vi "OFBS_readTrainingData.vi"(6 "Use equal number of trials?":bool, 8 "error in (no error)":errorcluster, 9 "ControlRefs":T1, 10 "NumberOfChannels":i32, 11 "OFBS class in":refnum<class "OptFreqBandsSearch.lvclass">) -> (0 "error out":errorcluster, 2 "Num of Trials of each Class":i32[](array[numeric]), 3 "OFBS class out":refnum<class "OptFreqBandsSearch.lvclass">)   [LabVIEW 2016, in "Optimal Frequency Bands Search.lvlib" / "OptFreqBandsSearch.lvclass"]
doc: "Метод, реализующий чтение обучающих данных (проб) из xml файла"
uses:
  OptFreqBandsSearch.lvclass
  OptFreqBandsSearch.lvclass/OptFreqBandsSearch.ctl
  <vilib>/xml/Load XML File.vi
  <vilib>/xml/Close Reference(Node).vi
  _XML_EEG_Features/XML_EEG_Features.lvlib
  <vilib>/xml/NI_XML.lvlib
  Optimal Frequency Bands Search.lvlib
panel:
  # "This VI is a part of BCI Design library, http://www.ru-bci.org \nCopyright © 2020, Sotnikov Peter, All rights reserved. License: GNU GPLv3"
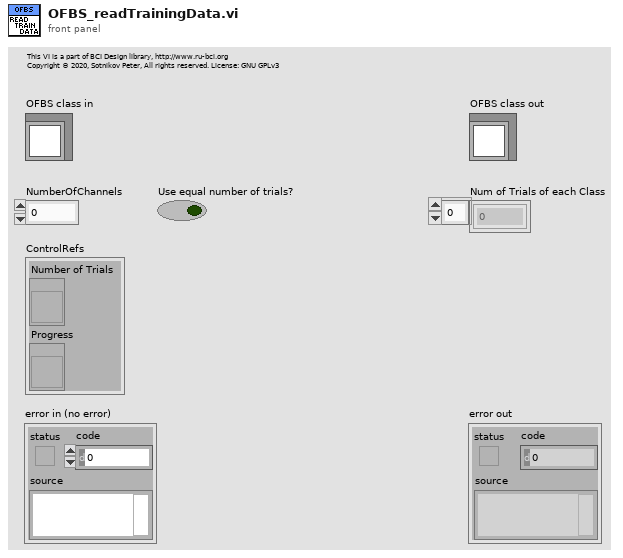
[diagram p1: front panel]
types:
  T1 = cluster{"Number of Trials":refnum<vi>, "Progress":refnum<vi>}
  T2 = typedef "XML_EEG_Features.lvlib/XML_FF_Header.ctl" = cluster{"NumberOfTrials":i32, "NumberOfClasses":i32, "FeatureVectorLength":i32, "FeatureExtractionMethod":string}
  T3 = typedef "XML_EEG_Features.lvlib/XML_FF_Trial.ctl" = cluster{"ClassLabel":string, "FeatureVector":dbl[]}
  T4 = cluster{"ClassLabel":string, "FeatureVector":dbl[][]}
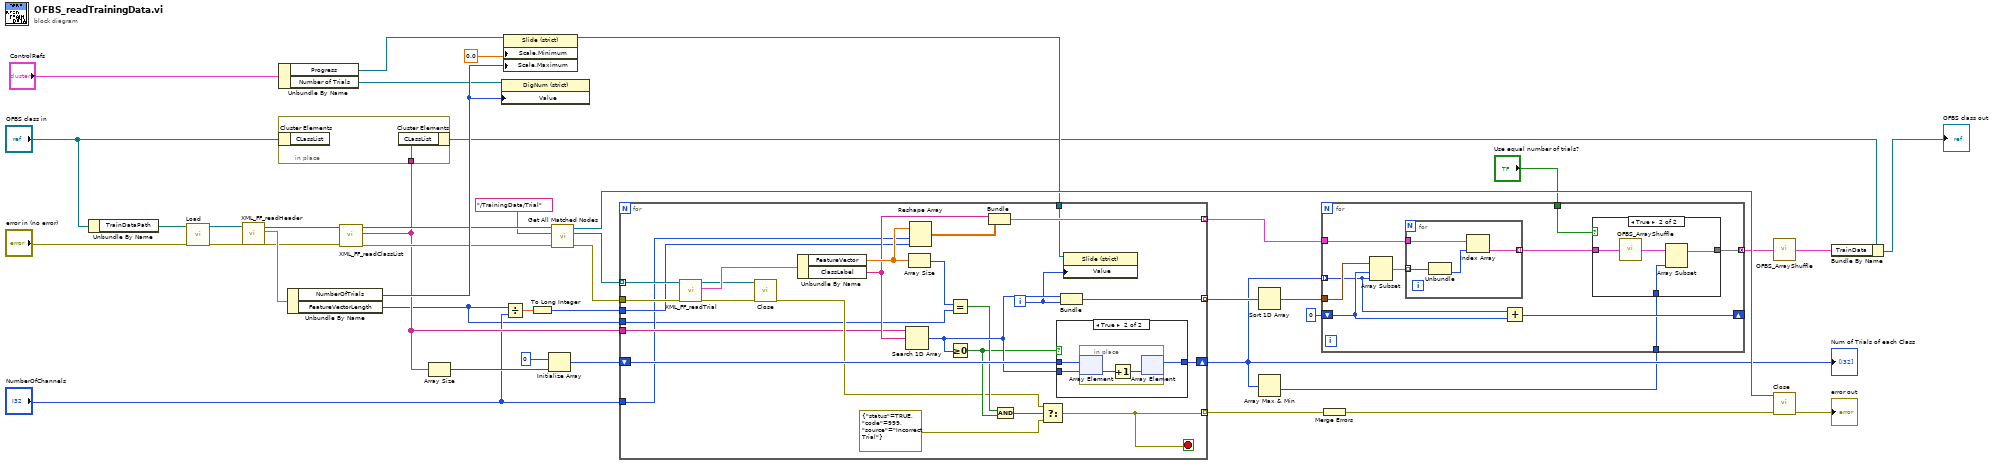
[diagram p0: block diagram]
diagram:
  n1 = Unbundle By Name("OFBS class in") -> ("TrainDataPath"=w42:path)
  n2 = call-poly <vilib>:"Load.vi"("path to XML document"=w42, "error in (no error)"="error in (no error)") -> ("DOM document out"=w39:refnum<k20>, "error out"=w40:errorcluster)  [unwired: 11 in, 1 out]
  n3 = call "XML_FF_readHeader.vi"("error in (no error)"=w40, "DOM document in"=w39) -> ("error out"=w31:errorcluster, "FF_Header out"=w38:T2, "DOM document out"=w32:refnum<k20>)  [unwired: 7 in]
  n4 = Unbundle By Name("ControlRefs") -> ("Progress"=w12:refnum<vi>, "Number of Trials"=w11:refnum<vi>)
  n5 = Unbundle By Name(w38) -> ("NumberOfTrials"=w34:i32, "FeatureVectorLength"=w8:i32)
  n6 = call "XML_FF_readClassList.vi"("error in (no error)"=w31, "DOM document in"=w32) -> ("error out"=w28:errorcluster, "CLassLabels out"=w15:string[], "DOM document out"=w29:refnum<k20>)  [unwired: 7 in]
  n7 = in-place "In Place Element Structure" {
    in-place-border: w15 -> [w43]
    n8 = in-place-cluster #1("OFBS class in") -> ()  [unwired: 1 out]
    n9 = in-place-cluster #1("CLassList"=w43) -> (w3:refnum<class "OptFreqBandsSearch.lvclass">)
  }
  n10 = Array Size(array=w15) -> (size(s)=w14:i32)
  n11 = property class="DigNum (strict)"(reference=w11, "Value"=w34) -> ()  [unwired: 1 in, 2 out]
  n12 = property class="Slide (strict)"(reference=w12, "Scale.Minimum"=0.0 ("Data Entry Limits:Minimum"), "Scale.Maximum"=w34) -> (reference out=w13:refnum<vi>)  [unwired: 1 in, 1 out]
  n13 = Divide(x=w8, y="NumberOfChannels") -> (x/y=w36:dbl)
  n14 = To Long Integer(number=w36) -> (32bit integer=w10:i32)
  n15 = Initialize Array(0, w14) -> (w25:i32[])
  n16 = call <vilib>:"Get All Matched Nodes.vi"("error in (no error)"=w28, "XPath expression"="/TrainingData/Trial", "node in"=w29) -> ("error out"=w16:errorcluster, "node result array"=w17:refnum<k20>[], "node out"=w27:refnum<k20>)  [unwired: 6 in]
  n17 = for {
    tunnel: [w56] -> w7 mode=indexing
    tunnel: [w52] -> w22 mode=indexing
    shift-right: [w63] -> w19
    shift-left: w25 -> [w64]
    tunnel: [w62] -> w21 mode=indexing
    tunnel: w17 -> [w50] mode=indexing
    tunnel: w16 -> [w49]
    tunnel: w15 -> [w48]
    tunnel: w13 -> [w47]
    tunnel: w10 -> [w46]
    tunnel: "NumberOfChannels" -> [w45]
    tunnel: w8 -> [w44]
    i -> [w51]
    stop <- w56 stop-if-true
    n18 = call "XML_FF_readTrial.vi"("error in (no error)"=w49, "DOM document in"=w50) -> ("error out"=w66:errorcluster, "Trial out"=w68:T3, "DOM document out"=w65:refnum<k20>)  [unwired: 7 in]
    n19 = call-poly <vilib>:"Close.vi"("error in (no error)"=w66, "node"=w65) -> ("error out"=w57:errorcluster)  [unwired: 7 in]
    n20 = Unbundle By Name(w68) -> ("FeatureVector"=w55:dbl[], "ClassLabel"=w54:string)
    n21 = Search 1D Array(1D array=w48, element=w54) -> (index of element=w61:i32)  [unwired: 1 in]
    n22 = Array Size(array=w55) -> (size(s)=w69:i32)
    n23 = Reshape Array(w55, w45, w46) -> (w53:dbl[][])
    n24 = Equal?(x=w69, y=w44) -> (x = y?=w60:bool)
    n25 = Greater Or Equal To 0?(x=w61) -> (x >= 0?=w59:bool)
    n26 = Bundle("ClassLabel"=w54, "FeatureVector"=w53) -> (w52:T4)  [unwired: 1 in]
    n27 = And(x=w60, y=w59) -> (x .and. y?=w58:bool)
    n28 = Select(t=w57, s=w58, f=errorcluster {"status"=TRUE, "code"=999, "source"="Incorrect Trial"} ("error out")) -> (s? t:f=w56:errorcluster)
    n29 = case shown="True" w59 {
      tunnel: w64 -> [w70 w73]
      tunnel: [w70 w72] -> w63
      tunnel: w61 -> [_ w71]
      frame False {
      }
      frame True {
        n30 = in-place {
          n31 = in-place-array #2(w73, w71) -> (w75:i32)
          n32 = Increment(x=w75) -> (x+1=w74:i32)
          n33 = in-place-array #2(w74) -> (w72:i32[])  [unwired: 1 out]
        }
      }
    }
    n34 = Bundle("index of element"=w61, w51) -> (w62:cluster{"index of element":i32, i32})  [unwired: 1 in]
    n35 = property class="Slide (strict)"(reference=w47, "Value"=w51) -> ()  [unwired: 1 in, 2 out]
  }
  "Num of Trials of each Class" <- w19
  n36 = Sort 1D Array(array=w21) -> (sorted array=w20:cluster{"index of element":i32, i32}[])
  n37 = Array Max & Min(array=w19) -> (min value=w18:i32)  [unwired: 3 out]
  n38 = for {
    tunnel: w19 -> [w80] mode=indexing
    tunnel: w20 -> [w84]
    tunnel: w22 -> [w85]
    shift-right: [w82] -> _
    shift-left: 0 -> [w81]
    tunnel: w18 -> [w78]
    tunnel: [w77] -> w5 mode=concatenating
    tunnel: "Use equal number of trials?" -> [w76]
    n39 = Array Subset(array=w84, index=w81, length=w80) -> (w83:cluster{"index of element":i32, i32}[])
    n40 = for {
      tunnel: w83 -> [w94] mode=indexing
      tunnel: [w92] -> w79 mode=indexing
      tunnel: w85 -> [w91]
      n41 = Unbundle(w94) -> (w93:i32)  [unwired: 1 out]
      n42 = Index Array(array=w91, index=w93) -> (element=w92:T4)
    }
    n43 = Add(x=w80, y=w81) -> (x+y=w82:i32)
    n44 = case shown="True" w76 {
      tunnel: w79 -> [w86 w89]
      tunnel: w78 -> [_ w90]
      tunnel: [w86 w87] -> w77
      frame False {
      }
      frame True {
        n45 = call "OFBS_ArrayShuffle.vi"("Array in"=w89) -> ("Array out"=w88:cluster{"ClassLabel":string, "Trial":dbl[][]}[])
        n46 = Array Subset(array=w88, length=w90) -> (w87:cluster{"ClassLabel":string, "Trial":dbl[][]}[])  [unwired: 1 in]
      }
    }
  }
  n47 = Merge Errors(w7) -> (w6:errorcluster)
  n48 = call "OFBS_ArrayShuffle.vi"("Array in"=w5) -> ("Array out"=w2:cluster{"ClassLabel":string, "Trial":dbl[][]}[])
  n49 = call-poly <vilib>:"Close.vi"("error in (no error)"=w6, "node"=w27) -> ("error out"=→"error out":errorcluster)  [unwired: 7 in]
  n50 = Bundle By Name(cluster=w3, "TrainData"=w2) -> (→"OFBS class out":refnum<class "OptFreqBandsSearch.lvclass">)
